vi "tempControl.vi"() -> ()   [LabVIEW 2018]
panel:
  out "FAN SPEED":dbl(knob) scale=0.0..5.0 scale format="%#_6f"
  out "FAN ON":bool
  out "HEATER  ON":bool
  out "COOLER ON":bool
  out "Thermometer":dbl(slide) scale=-10.0..60.0
  out "HIGH\nTEMP":bool
  out "LOW\nTEMP":bool
  out "MEDIUM \nTEMP":bool
  in  "INPUT TEMERATURE \n                 KNOB":dbl(knob) scale=-10.0..60.0
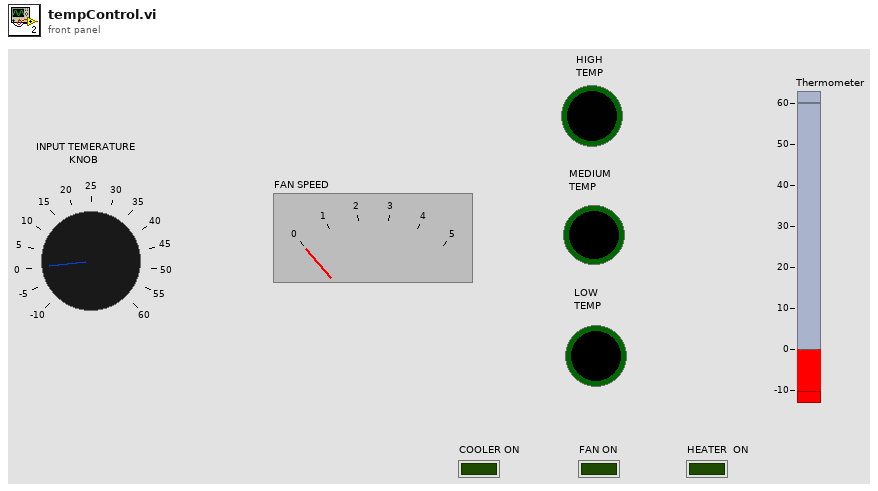
[diagram p1: front panel]
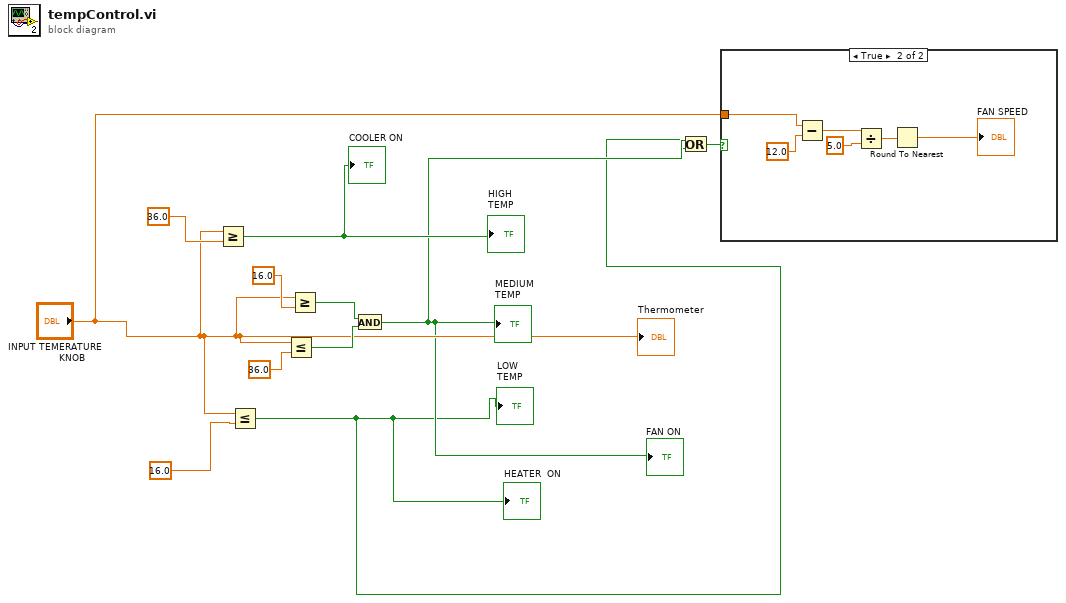
[diagram p0: block diagram]
diagram:
  n1 = Greater Or Equal?(x="INPUT TEMERATURE \n                 KNOB", y=36.0 ("x")) -> (x >= y?=→"HIGH\nTEMP" →"COOLER ON":bool)
  n2 = Less Or Equal?(x="INPUT TEMERATURE \n                 KNOB", y=16.0) -> (x <= y?=w2:bool)
  "LOW\nTEMP" <- w2
  "HEATER  ON" <- w2
  n3 = Less Or Equal?(x="INPUT TEMERATURE \n                 KNOB", y=36.0 ("x")) -> (x <= y?=w9:bool)
  n4 = Greater Or Equal?(x="INPUT TEMERATURE \n                 KNOB", y=16.0 ("x")) -> (x >= y?=w10:bool)
  n5 = And(x=w10, y=w9) -> (x .and. y?=w3:bool)
  "MEDIUM \nTEMP" <- w3
  "FAN ON" <- w3
  n6 = Or(x=w3, y=w2) -> (x .or. y?=w1:bool)
  n7 = case shown="True" w1 {
    tunnel: "INPUT TEMERATURE \n                 KNOB" -> [_ w12]
    frame False {
    }
    frame True {
      n8 = Subtract(x=w12, y=12.0) -> (x-y=w17:dbl)
      n9 = Divide(x=w17, y=5.0) -> (x/y=w15:dbl)
      n10 = Round To Nearest(number=w15) -> (nearest integer value=→"FAN SPEED":dbl)
    }
  }
  "Thermometer" <- "INPUT TEMERATURE \n                 KNOB"
